vi "HandleTrigger.vi"(8 "error in (no error)":errorcluster, 9 "Current Trigger Value":dbl, 10 "Previous Trigger Value":dbl, 11 "Channel Manager in":refnum<class "Channel Manager.lvclass">) -> (0 "error out":errorcluster, 3 "Channel Manager out":refnum<class "Channel Manager.lvclass">)   [LabVIEW 2024, in "Embedded TDMS Logger Engine.lvlib" / "Channel Manager.lvclass"]
doc: "Overall handler of the trigger, calculates the logic of the trigger state and then if just triggered - opens a new file, if just \"untriggered\", close the file. Log the trigger state and last value for the next stage and iteration.s"
uses:
  Channel Manager.lvclass
  Channel Manager.lvclass/Channel Manager.ctl
  Shared/File Classes/File/File.lvclass
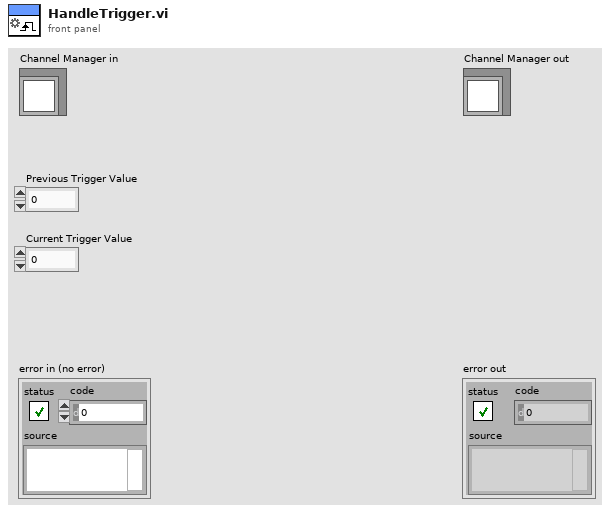
[diagram p1: front panel]
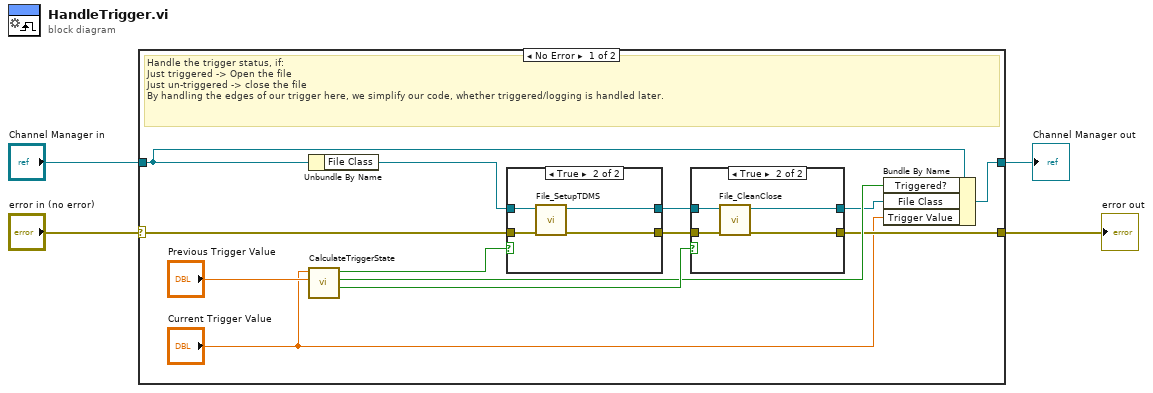
[diagram p0: block diagram]
diagram:
  n1 = case shown="No Error" "error in (no error)" {
    selector: "error in (no error)" -> [w13 w31]
    tunnel: [w7 w31] -> w3
    tunnel: [w11 w30] -> w1
    tunnel: "Channel Manager in" -> [w15 w30]
    frame No Error {
      # "Handle the trigger status, if:\nJust triggered -> Open the file\nJust un-triggered -> close the file\nBy handling the edges of our trigger here, we simplify our code, whether triggered/logging is handled later."
      n2 = Unbundle By Name(w15) -> ("File Class"=w14:refnum<class "File.lvclass">)
      n3 = call "CalculateTriggerState.vi"("Previous Trigger Value"="Previous Trigger Value", "Current Trigger Value"="Current Trigger Value") -> ("End Triggered/Close?"=w12:bool, "Triggered/Logging?"=w10:bool, "Just Triggered/Setup?"=w16:bool)  [unwired: 7 in]
      n4 = case shown="True" w16 {
        tunnel: w14 -> [w25 w29]
        tunnel: w13 -> [w24 w26]
        tunnel: [w24 w28] -> w9
        tunnel: [w25 w27] -> w8
        frame False {
        }
        frame True {
          n5 = call-dynamic "File_SetupTDMS.vi"("error in (no error)"=w26, "File in"=w29) -> ("error out"=w28:errorcluster, "File out"=w27:refnum<class "File.lvclass">)  [unwired: 8 in]
        }
      }
      n6 = case shown="True" w12 {
        tunnel: w9 -> [w19 w22]
        tunnel: w8 -> [w18 w23]
        tunnel: [w19 w21] -> w7
        tunnel: [w18 w20] -> w6
        frame False {
        }
        frame True {
          n7 = call-dynamic "File_CleanClose.vi"("error in (no error)"=w22, "File in"=w23) -> ("error out"=w21:errorcluster, "File out"=w20:refnum<class "File.lvclass">)  [unwired: 8 in]
        }
      }
      n8 = Bundle By Name(cluster=w15, "Triggered?"=w10, "File Class"=w6, "Trigger Value"="Current Trigger Value") -> (w11:refnum<class "Channel Manager.lvclass">)
    }
    frame Error {
    }
  }
  "error out" <- w3
  "Channel Manager out" <- w1
